vi "Set Scheme.vi"(8 "error in (no error)":errorcluster, 10 "Scheme":string, 11 "Protocol Config in":refnum<class "Protocol Config.lvclass">) -> (0 "error out":errorcluster, 3 "Protocol Config out":refnum<class "Protocol Config.lvclass">)   [LabVIEW 2020, in "Examples.lvlib" / "Protocol Config.lvclass"]
uses:
  Protocol Config.lvclass
  Protocol Config.lvclass/Protocol Config.ctl
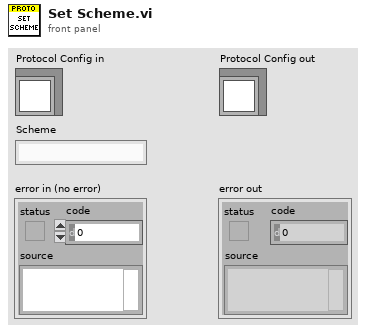
[diagram p1: front panel]
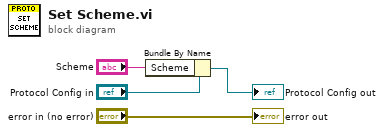
[diagram p0: block diagram]
diagram:
  n1 = Bundle By Name(cluster="Protocol Config in", "Scheme"="Scheme") -> (→"Protocol Config out":refnum<class "Protocol Config.lvclass">)
  "error out" <- "error in (no error)"
